vi "UUT Result With Print Option Dialog.vi"(8 "Max Retests":u8, 9 "Failed Test Counter":u8, 10 "Select Dialog":T2(ring)=enum."Failed") -> (2 "Print Current Report?":bool, 3 "OK Button Text Out":string)   [LabVIEW 2010]
uses:
  _TypeDefs/OK Button_TouchScreen.ctl
panel:
  in  "The Print button is moved off of the visible front pael \nbecause the decision was made to move all functionality\nof the print function into the report generation code.":T1
  out "Message":string
  in  "OK":T1
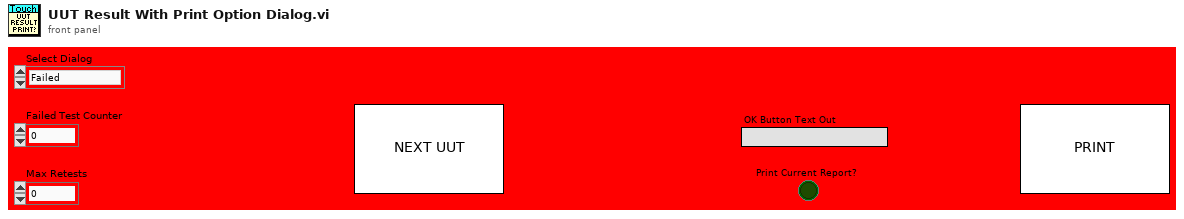
[diagram p1: front panel]
types:
  T1 = typedef "OK Button_TouchScreen.ctl" = bool
  T2 = enum16{"Passed", "Failed", "Error", "Terminated"}
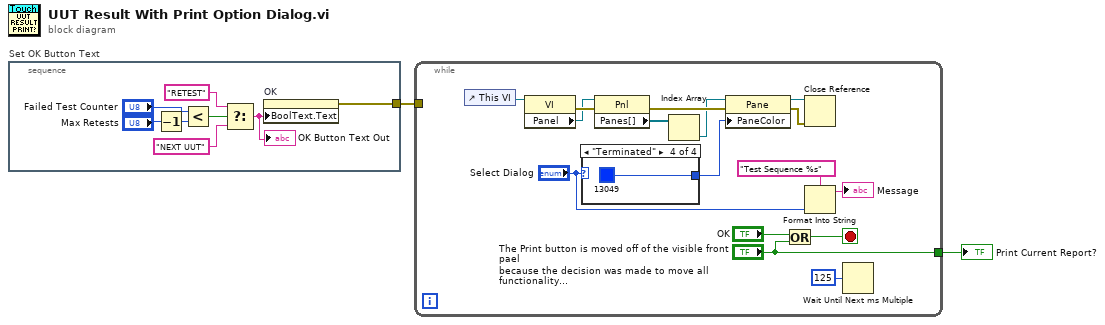
[diagram p0: block diagram]
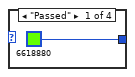
[diagram p2: hidden frame]
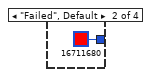
[diagram p3: hidden frame]
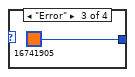
[diagram p4: hidden frame]
diagram:
  n1 = stacked-sequence "Set OK Button Text" {
    tunnel: [w6] -> w2
    frame #0 {
      n2 = Decrement(x="Max Retests") -> (x-1=w3:u8)
      n3 = Less?(x="Failed Test Counter", y=w3) -> (x < y?=w8:bool)
      n4 = Select(t="RETEST", s=w8, f="NEXT UUT") -> (s? t:f=w5:string)
      "OK Button Text Out" <- w5
      n5 = property on="OK" class="Bool"("BoolText.Text"=w5) -> (error out=w6:errorcluster)  [unwired: 2 in, 1 out]
    }
  }
  n6 = while {
    tunnel: w2 -> [_]
    tunnel: ["The Print button is moved off of the visible front pael \nbecause the decision was made to move all functionality\nof the print function into the report generation code."] -> w1
    stop <- w12 stop-if-true
    n7 = control-ref of="This VI"() -> (w13:refnum<vi>)
    n8 = property class="VI"(reference=w13) -> (error out=w20:errorcluster, "Panel"=w19:refnum<vi>)  [unwired: 1 in, 1 out]
    n9 = case shown="\"Terminated\"" "Select Dialog" {
      tunnel: [u32 6618880 u32 16711680 u32 16741905 u32 13049] -> w14
      frame "Passed" {
      }
      frame "Failed", Default {
      }
      frame "Error" {
      }
      frame "Terminated" {
      }
    }
    n10 = property class="Pnl"(reference=w19, error in=w20) -> (error out=w18:errorcluster, "Panes[]"=w21:refnum<vi>[])  [unwired: 1 out]
    n11 = Index Array(array=w21) -> (element=w17:refnum<vi>)  [unwired: 1 in]
    n12 = property class="Pane"(reference=w17, error in=w18, "PaneColor"=w14) -> (reference out=w16:refnum<vi>, error out=w15:errorcluster)
    n13 = Or(x="OK", y="The Print button is moved off of the visible front pael \nbecause the decision was made to move all functionality\nof the print function into the report generation code.") -> (x .or. y?=w12:T1)
    n14 = Close Reference(reference=w16, error in (no error)=w15) -> ()  [unwired: 1 out]
    n15 = Format Into String(format string="Test Sequence %s" ("Message"), "Select Dialog") -> (resulting string=→"Message":string)  [unwired: 2 in, 1 out]
    n16 = Wait Until Next ms Multiple(millisecond multiple=u32 125) -> ()  [unwired: 1 out]
  }
  "Print Current Report?" <- w1
